vi "Set output state.vi"(8 "error in":errorcluster, 10 "Output state":u16(ring) items=["0 - OFF", "1 - ON"], 11 "VISA resource name":refnum<visa-resource-name>) -> (0 "error out":errorcluster, 3 "VISA resource name out":refnum<visa-resource-name>)   [LabVIEW 2020, in "Datron D4xxx.lvlib"]
doc: "This VI changes state of output."
uses:
  Datron D4xxx.lvlib
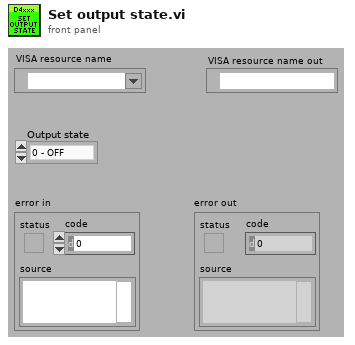
[diagram p1: front panel]
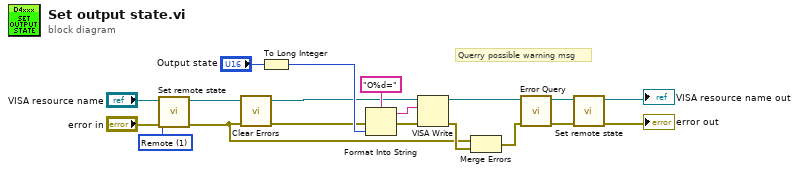
[diagram p0: block diagram]
diagram:
  w8 = u16 1 items=["Local", "Remote", "Default"] ("Remote state")
  # "Querry possible warning msg"
  n1 = call "Set remote state.vi"("error in"="error in", "Remote state"=w8, "VISA resource name"="VISA resource name") -> ("error out"=w1:errorcluster, "VISA resource name out"=w9:refnum<visa-resource-name>)  [unwired: 7 in]
  n2 = call <vilib>:"Clear Errors.vi"("error in (no error)"=w1) -> ("error out"=w4:errorcluster)  [unwired: 5 in, 1 out]
  n3 = To Long Integer(number="Output state") -> (32bit integer=w18:i32)
  n4 = Format Into String(format string="O%d=", error in=w4, w18) -> (resulting string=w16:string, error out=w15:errorcluster)  [unwired: 1 in]
  n5 = VISA Write(VISA resource name=w9, write buffer=w16, error in (no error)=w15) -> (VISA resource name out=w6:refnum<visa-resource-name>, error out=w3:errorcluster)  [unwired: 1 out]
  n6 = Merge Errors(w1, w3) -> (w2:errorcluster)
  n7 = call "Error Query.vi"("error in (no error)"=w2, "VISA resource name"=w6) -> ("error out"=w7:errorcluster, "VISA resource name out"=w5:refnum<visa-resource-name>)  [unwired: 6 in, 2 out]
  n8 = call "Set remote state.vi"("error in"=w7, "VISA resource name"=w5) -> ("error out"=→"error out":errorcluster, "VISA resource name out"=→"VISA resource name out":refnum<visa-resource-name>)  [unwired: 8 in]
